vi "模块启用配置框.vi"() -> ()   [LabVIEW 2016]
uses:
  <vilib>/Utility/config.llb/NI_LVConfig.lvlib
panel:
  in  "总氮启用":bool caption="总磷总氮禁用"
  in  "超标留样启用":bool caption="流量计禁用"
  in  "取消":bool
  in  "确认":bool
  in  "CODMn启用":bool caption="CODMn禁用"
  in  "质控单元启用":bool caption="质控单元禁用"
  in  "总磷启用":bool caption="总磷总氮禁用"
  in  "流量计启用":bool caption="流量计禁用"
  in  "氨氮启用":bool caption="氨氮禁用"
  in  "多参数启用":bool caption="多参数禁用"
  in  "CODcr启用":bool caption="CODcr禁用"
  # "模块启用配置"
  # "说明:\n选择所需要启动的模块,并按确认,软件将重启生效."
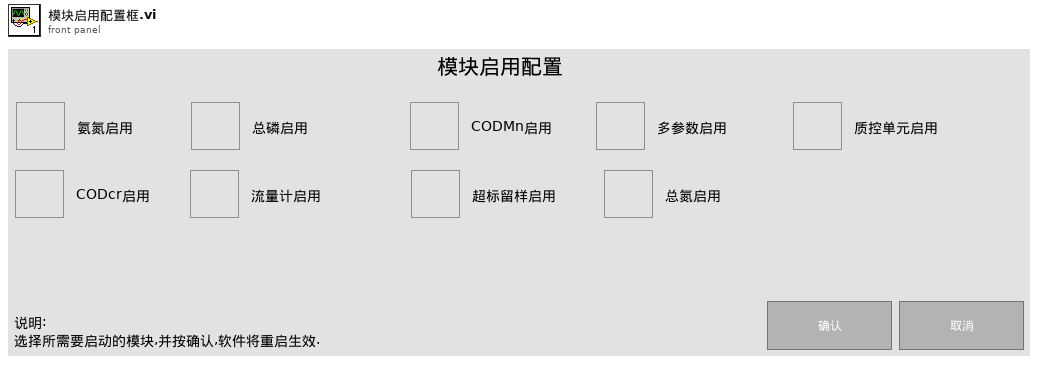
[diagram p1: front panel]
types:
  T1 = typedef "NI_LVConfig.lvlib/Config Data RefNum.ctl" = refnum<k1>
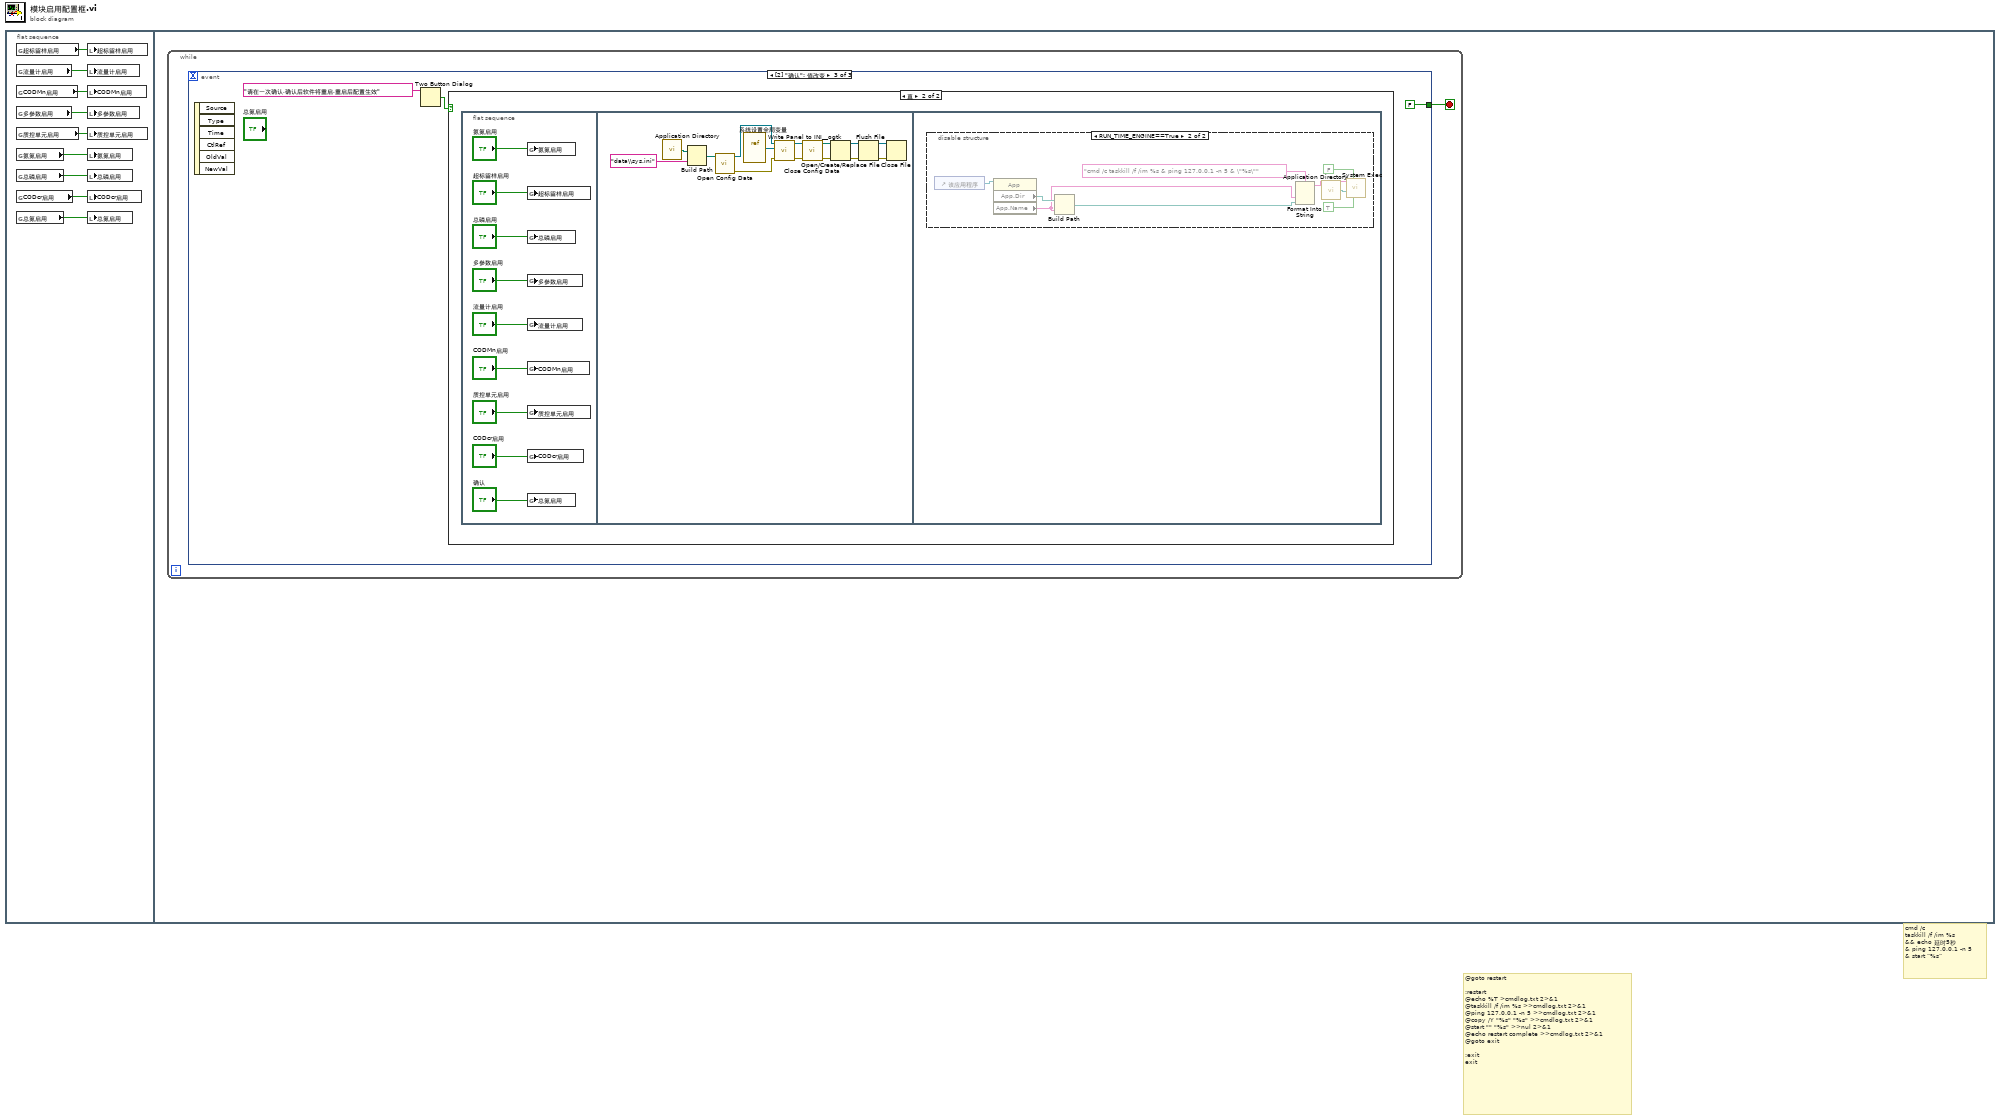
[diagram p0: block diagram]
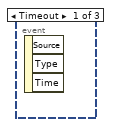
[diagram p2: hidden frame]
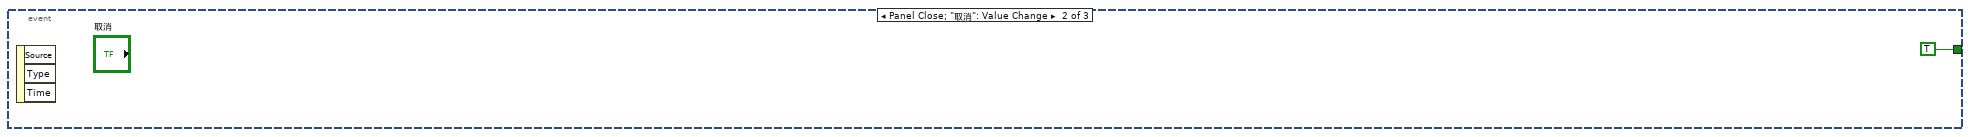
[diagram p3: hidden frame]
diagram:
  # "@goto restart\n\n:restart\n@echo %T >cmdlog.txt 2>&1\n@taskkill /f /im %s >>cmdlog.txt 2>&1\n@ping 127.0.0.1 -n 5 >>cmdlog.txt 2>&1\n@copy /Y \"%s\" \"%s\" >>cmdlog.txt 2>&1\n@start \"\" \"%s\" >>nul 2>&1\n@echo restart complete >>cmdlog.txt 2>&1\n@goto exit\n\n:exit\nexit"
  # "cmd /c\ntaskkill /f /im %s \n&& echo 延时5秒 \n& ping 127.0.0.1 -n 5 \n& start “%s”"
  n1 = flat-sequence {
    frame #0 {
      n2 = global read "系统设置全局变量.vi" "超标留样启用"() -> (w2:bool)
      n3 = global read "系统设置全局变量.vi" "流量计启用"() -> (w6:bool)
      n4 = global read "系统设置全局变量.vi" "CODMn启用"() -> (w4:bool)
      n5 = global read "系统设置全局变量.vi" "多参数启用"() -> (w7:bool)
      n6 = global read "系统设置全局变量.vi" "质控单元启用"() -> (w3:bool)
      n7 = global read "系统设置全局变量.vi" "氨氮启用"() -> (w5:bool)
      n8 = global read "系统设置全局变量.vi" "总磷启用"() -> (w8:bool)
      n9 = global read "系统设置全局变量.vi" "CODcr启用"() -> (w9:bool)
      n10 = global read "系统设置全局变量.vi" "总氮启用"() -> (w1:bool)
      n11 = local write "超标留样启用"(w2) -> ()
      n12 = local write "流量计启用"(w6) -> ()
      n13 = local write "CODMn启用"(w4) -> ()
      n14 = local write "多参数启用"(w7) -> ()
      n15 = local write "质控单元启用"(w3) -> ()
      n16 = local write "氨氮启用"(w5) -> ()
      n17 = local write "总磷启用"(w8) -> ()
      n18 = local write "CODcr启用"(w9) -> ()
      n19 = local write "总氮启用"(w1) -> ()
    }
    frame #1 {
      n20 = while {
        stop <- w10 stop-if-true
        n21 = event shown="[2] \"确认\": 值改变" {
          selector: _ -> [_ _ _]
          dyn-events: _ -> [_ _ _]
          timeout: _ -> [_ _ _]
          tunnel: [_ TRUE FALSE] -> w10
          event Timeout {
            n22 = event-data() -> ()  [unwired: 1 in, 3 out]
          }
          event Panel Close; "取消": Value Change {
            n23 = event-data() -> ()  [unwired: 1 in, 3 out]
          }
          event "确认": Value Change {
            n24 = event-data() -> ()  [unwired: 1 in, 6 out]
            n25 = Two Button Dialog(message="请在一次确认,确认后软件将重启,重启后配置生效" ("消息")) -> (T button?=w12:bool)  [unwired: 2 in]
            n26 = case shown="真" w12 {
              frame False {
              }
              frame True {
                n27 = flat-sequence {
                  frame #0 {
                    n28 = global write "系统设置全局变量.vi" "氨氮启用"("氨氮启用") -> ()
                    n29 = global write "系统设置全局变量.vi" "超标留样启用"("超标留样启用") -> ()
                    n30 = global write "系统设置全局变量.vi" "总磷启用"("总磷启用") -> ()
                    n31 = global write "系统设置全局变量.vi" "多参数启用"("多参数启用") -> ()
                    n32 = global write "系统设置全局变量.vi" "流量计启用"("流量计启用") -> ()
                    n33 = global write "系统设置全局变量.vi" "CODMn启用"("CODMn启用") -> ()
                    n34 = global write "系统设置全局变量.vi" "质控单元启用"("质控单元启用") -> ()
                    n35 = global write "系统设置全局变量.vi" "CODcr启用"("CODcr启用") -> ()
                    n36 = global write "系统设置全局变量.vi" "总氮启用"("确认") -> ()
                  }
                  frame #1 {
                    n37 = call <vilib>:"Application Directory.vi"() -> ("Application Directory"=w37:path)
                    n38 = Build Path(base path=w37, name or relative path="data\\sys.ini" ("名称或相对路径")) -> (appended path=w35:path)
                    n39 = call <vilib>:"Open Config Data.vi"("configuration file path"=w35) -> ("error out"=w31:errorcluster, "refnum"=w34:T1)  [unwired: 8 in, 1 out]
                    n40 = vi-ref "系统设置全局变量.vi"() -> (w33:refnum<vi>)
                    n41 = call <userlib>:"Write Panel to INI__ogtk.vi"("error in (no error)"=w31, "VI ref"=w33, "refnum"=w34) -> ("error out"=w30:errorcluster, "refnum out"=w32:T1)  [unwired: 7 in]
                    n42 = call <vilib>:"Close Config Data.vi"("error in (no error)"=w30, "refnum"=w32) -> ("error out"=w25:errorcluster, "file path"=w24:path)  [unwired: 8 in]
                    n43 = Open/Create/Replace File(file path (use dialog)=w24, error in=w25) -> (refnum out=w28:refnum<file>, error out=w29:errorcluster)  [unwired: 4 in, 1 out]
                    n44 = Flush File(refnum=w28, error in=w29) -> (refnum out=w27:refnum<file>, error out=w26:errorcluster)
                    n45 = Close File(refnum=w27, error in=w26) -> ()  [unwired: 2 out]
                  }
                  frame #2 {
                    n46 = disable-structure shown="RUN_TIME_ENGINE==True" {
                      frame condition #0 (active) {
                      }
                      frame condition #1 {
                        n47 = control-ref of="该应用程序"() -> (w46:refnum<vi>)
                        n48 = property class="App"(reference=w46) -> ("App.Dir"=w42:path, "App.Name"=w41:string)  [unwired: 1 in, 2 out]
                        n49 = Build Path(base path=w42, name or relative path=w41) -> (appended path=w40:path)
                        n50 = Format Into String(format string="cmd /c taskkill /f /im %s & ping 127.0.0.1 -n 5 & \"%s\"" ("格式字符串"), w41, w40) -> (resulting string=w44:string)  [unwired: 2 in, 1 out]
                        n51 = call <vilib>:"Application Directory.vi"() -> ("Application Directory"=w43:path)
                        n52 = call <vilib>:"System Exec.vi"("run minimized? (F)"=TRUE, "wait until completion? (T)"=FALSE, "working directory"=w43, "command line"=w44) -> ()  [unwired: 4 in, 4 out]
                      }
                    }
                  }
                }
              }
            }
          }
        }
      }
    }
  }
